vi "sub2.vi"() -> ()   [LabVIEW 2018]
uses:
  global_variable.vi
panel:
  out "숫자형 인디케이":dbl
  in  "정지버튼":bool
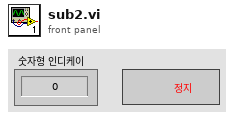
[diagram p1: front panel]
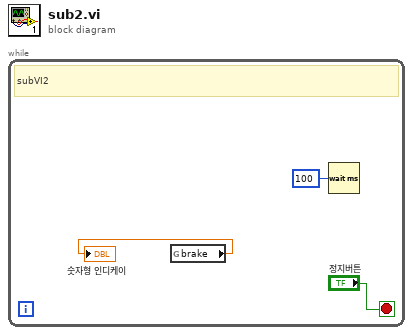
[diagram p0: block diagram]
diagram:
  n1 = while {
    stop <- "정지버튼" stop-if-true
    # "subVI2"
    n2 = global read "global_variable.vi" "brake"() -> (→"숫자형 인디케이":dbl)
    n3 = Wait (ms)(milliseconds to wait=u32 100 ("대기 시간 (ms)")) -> ()  [unwired: 1 out]
  }
